vi "get x And y As Point (I32).vi"(11 "Vector 2D in":refnum<class "Vector 2D.lvclass">) -> (3 "Point":T1)   [LabVIEW 2015, in "Vector 2D.lvclass"]
uses:
  Vector 2D.lvclass
  LabSDL2/Source/Libraries/SDL2 Utility/Point (I32).ctl
  Vector 2D.lvclass/Vector 2D.ctl
  LabSDL2/Source/Libraries/SDL2 Utility/SDL2 Utility.lvlib
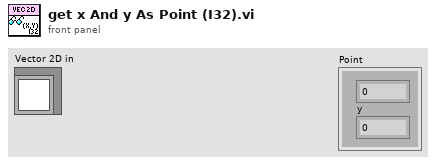
[diagram p1: front panel]
types:
  T1 = typedef "SDL2 Utility.lvlib/Point (I32).ctl" = cluster{"x":i32, "y":i32}
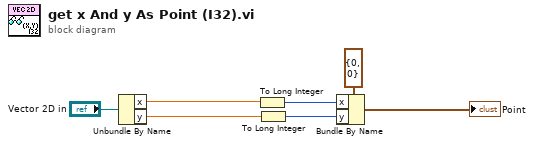
[diagram p0: block diagram]
diagram:
  n1 = Unbundle By Name("Vector 2D in") -> ("x"=w4:sgl, "y"=w2:sgl)
  n2 = To Long Integer(number=w4) -> (32bit integer=w3:i32)
  n3 = To Long Integer(number=w2) -> (32bit integer=w1:i32)
  n4 = Bundle By Name(cluster=T1 {"x"=0, "y"=0} ("Point"), "x"=w3, "y"=w1) -> (→"Point":T1)
